vi "Desktop Main.vi"() -> ()   [LabVIEW 2019]
doc: "Demonstrates how to use network streams to pass data and commands between two running VIs. It displays waveform data that is received from the target VI and sends commands to update the frequency of the generated signal."
uses:
  <vilib>/picture/3D Picture Control/NI_3D Picture Control.lvlib
  <resource>/objmgr/ni.dex.rc
panel:
  out "Ping B distance":dbl
  out "PING A distance":dbl
  out "connected?":bool
  in  "stop":bool
  out "myRIO Posture":refnum<vi>(3d-picture)
  in  "myRIO IP Address":string="172.22.11.2"
  # "Overview: This example can view myRIO posture that is estimated by RT Main.vi running on the myRIO device.\nRequirements: Network Streams on NI myRIO\nInstructions:\n1. Configure myRIO IP Address.\n2. Run RT Main.vi on the myRIO target.\n3. Run this VI."
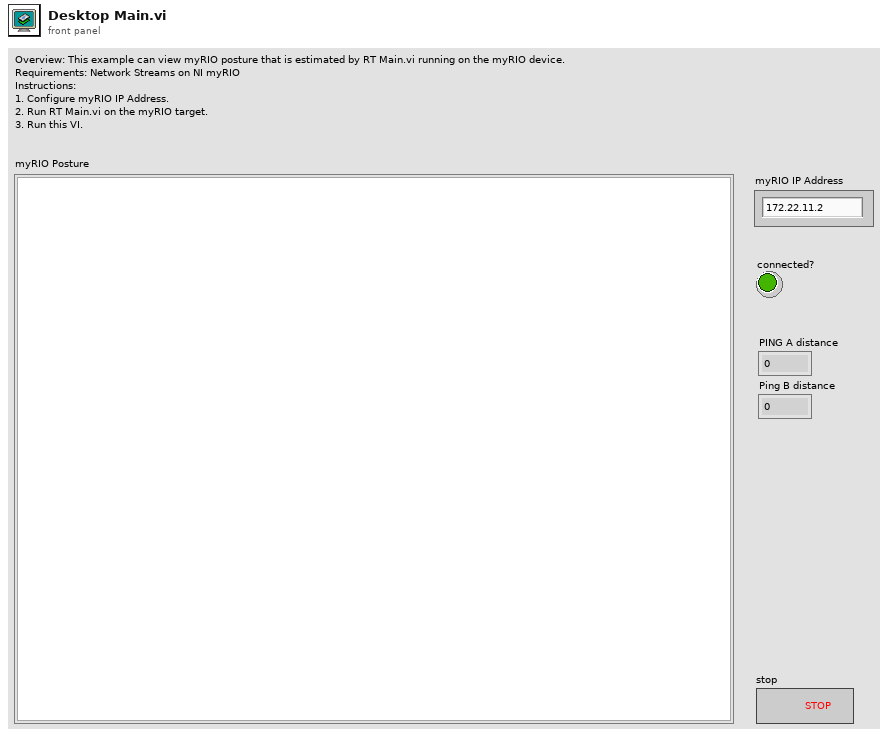
[diagram p1: front panel]
types:
  T1 = typedef "ROVdataOut.ctl" = cluster{"Rotation Angle":dbl, "Rotation Vector":cluster{"x":dbl, "y":dbl, "z":dbl}, "PING A distance":dbl, "Ping B distance":dbl, "angles":cluster{"roll":dbl, "pitch":dbl, "yaw":dbl}}
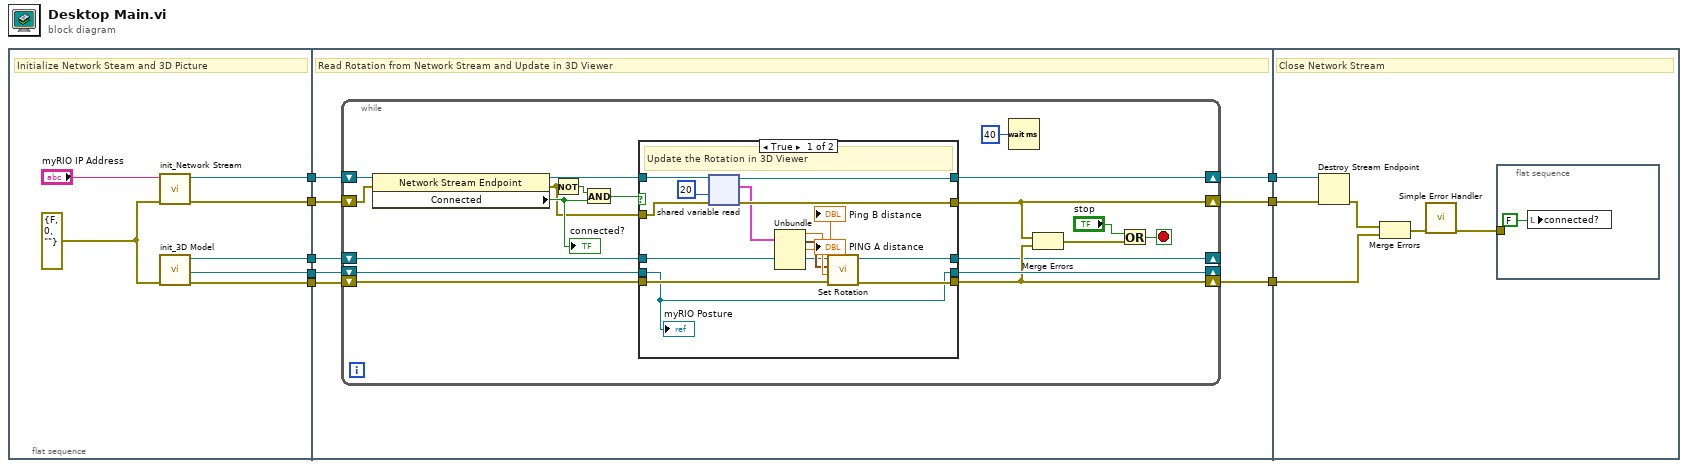
[diagram p0: block diagram]
diagram:
  n1 = flat-sequence {
    tunnel: [w14] -> w6
    tunnel: [w13] -> w5
    tunnel: [w12] -> w4
    tunnel: [w10] -> w3
    tunnel: [w9] -> w1
    tunnel: [w23] -> w8
    tunnel: [w22] -> w7
    tunnel: w6 -> [w21]
    tunnel: w5 -> [w20]
    tunnel: w4 -> [w19]
    tunnel: w3 -> [w18]
    tunnel: [w17] -> w2
    tunnel: w1 -> [w16]
    tunnel: w8 -> [w68]
    tunnel: w7 -> [w67]
    tunnel: w2 -> [w66]
    frame #0 {
      w11 = errorcluster {"status"=FALSE, "code"=0, "source"=""} ("error in")
      # "Initialize Network Steam and 3D Picture"
      n2 = call "init_Network Stream.vi"("error in"=w11, "MyRIO IP Address"="myRIO IP Address") -> ("error out"=w13:errorcluster, "reader"=w14:refnum<k21>)  [unwired: 8 in]
      n3 = call "init_3D Model.vi"("error in"=w11) -> ("error out"=w12:errorcluster, "Scene Object Out"=w10:refnum<vi>, "myRIO ref"=w9:refnum<vi>)  [unwired: 8 in]
    }
    frame #1 {
      # "Read Rotation from Network Stream and Update in 3D Viewer"
      n4 = while "Target->Host Data Reader" {
        shift-right: [w38] -> w22
        shift-left: w20 -> [w31]
        shift-right: [w40] -> w23
        shift-left: w21 -> [w32]
        shift-right: [w42] -> _
        shift-left: w18 -> [w41]
        shift-right: [w37] -> w17
        shift-left: w19 -> [w39]
        shift-right: [w24] -> _
        shift-left: w16 -> [w25]
        stop <- w36 stop-if-true
        n5 = property class="Network Stream Endpoint"(reference=w32, error in=w31) -> (reference out=w30:refnum<k21>, error out=w26:errorcluster, "Connected"=w28:bool)
        "connected?" <- w28
        n6 = Not(x=w26) -> (.not. x?=w29:bool)
        n7 = And(x=w29, y=w28) -> (x .and. y?=w27:bool)
        n8 = case shown="True" w27 {
          tunnel: [w55 w59] -> w38
          tunnel: w41 -> [w45 w62]
          tunnel: [w45 w62] -> w42
          tunnel: [w52 w60] -> w40
          tunnel: w39 -> [w47 w61]
          tunnel: [w48 w61] -> w37
          tunnel: w30 -> [w53 w60]
          tunnel: w26 -> [w51 w59]
          tunnel: w25 -> [w49 w58]
          tunnel: [w46 w58] -> w24
          frame True {
            # "Update the Rotation in 3D Viewer"
            n9 = shared-variable-read(w53, w51, 20 ("timeout ms")) -> (w52:refnum<k21>, w55:errorcluster, w54:T1)  [unwired: 1 out]
            n10 = Unbundle(w54) -> ("Rotation Angle"=w57:dbl, "Rotation Vector"=w56:cluster{"x":dbl, "y":dbl, "z":dbl}, "PING A distance"=→"PING A distance":dbl, "Ping B distance"=→"Ping B distance":dbl)  [unwired: 1 out]
            n11 = call <vilib>:"Set Rotation.vi"("error in (no error)"=w47, "Angle"=w57, "Axis"=w56, "Scene Object"=w49) -> ("error out"=w48:errorcluster, "Rotated Scene Object"=w46:refnum<vi>)  [unwired: 6 in]
            "myRIO Posture" <- w45
          }
          frame False {
          }
        }
        n12 = Wait (ms)(milliseconds to wait=u32 40) -> ()  [unwired: 1 out]
        n13 = Merge Errors(w38, w37) -> (w34:errorcluster)
        n14 = Or(x="stop", y=w34) -> (x .or. y?=w36:bool)
      }
    }
    frame #2 {
      # "Close Network Stream"
      n15 = Destroy Stream Endpoint(8:w67, 11:w68) -> (0:w65:errorcluster)
      n16 = Merge Errors(w65, w66) -> (w64:errorcluster)
      n17 = call <vilib>:"Simple Error Handler.vi"("error in (no error)"=w64) -> ("error out"=w63:errorcluster)  [unwired: 4 in, 4 out]
      n18 = flat-sequence {
        tunnel: w63 -> [_]
        frame #0 {
          n19 = local write "connected?"(FALSE) -> ()
        }
      }
    }
  }
